vi "Init Device List.vi"(8 "error in (no error)":errorcluster, 9 "Active Devices":refnum<vi>, 10 "Subpanels' ref":refnum<vi>[](array[refnum])) -> (0 "error out":errorcluster, 2 "find list":string[](array[string]), 3 "Device List State out":T1)   [LabVIEW 2015]
uses:
  Device List State.ctl
  Device/Device.lvclass
  <vilib>/Instr/_visa.llb/VISA Find Search Mode.ctl
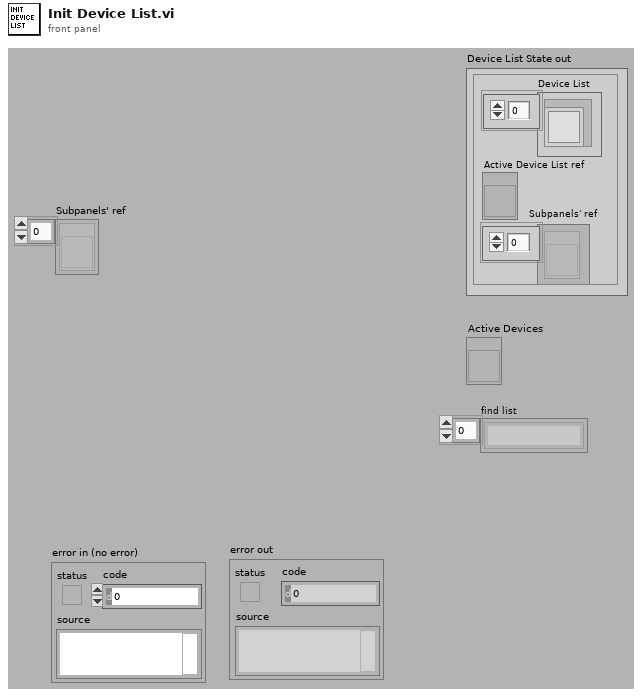
[diagram p1: front panel]
types:
  T1 = typedef "Device List State.ctl" = cluster{"Device List":refnum<class "Device.lvclass">[], "Active Device List ref":refnum<vi>, "Subpanels' ref":refnum<vi>[]}
  T2 = typedef "VISA Find Search Mode.ctl" = u32
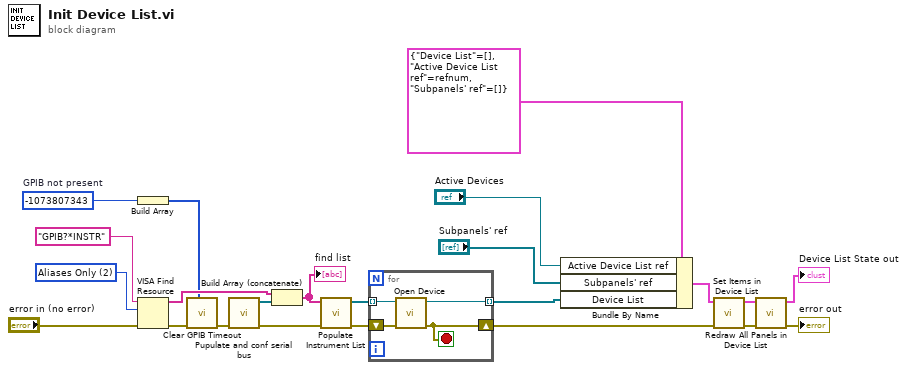
[diagram p0: block diagram]
diagram:
  w5 = -1073807343  # GPIB not present
  w22 = T2 2 items=["Canonical Names Only"=0, "Aliases Only"=2, "Include Matching Aliases"=3, "Include All Aliases"=4] ("Search Mode")
  n1 = Build Array(w5) -> (w4:i32[])
  n2 = VISA Find Resource(8:"error in (no error)", 10:w22, 11:"GPIB?*INSTR" ("expression (\"?*\")")) -> (0:w3:errorcluster, 3:w7:string[])  [unwired: 1 out]
  n3 = call "Clear GPIB Timeout.vi"("Errors to skip"=w4, "error in (no error)"=w3) -> ("error out"=w2:errorcluster)  [unwired: 9 out]
  n4 = call "Pupulate and conf serial bus.vi"("Error In"=w2) -> ("Error Out"=w1:errorcluster, "Devices"=w8:refnum<visa-resource-name>[])  [unwired: 9 in]
  n5 = Build Array (concatenate)(w7, w8) -> (w6:string[])
  "find list" <- w6
  n6 = call "Populate Instrument List.vi"("error in (no error)"=w1, "VISA Resourse Names"=w6) -> ("error out"=w20:errorcluster, "Instrument List"=w19:refnum<class "Instrument.lvclass">[])  [unwired: 2 in, 6 out]
  n7 = for {
    tunnel: w19 -> [w27] mode=indexing
    shift-right: [w24] -> w18
    shift-left: w20 -> [w25]
    tunnel: [w26] -> w11 mode=indexing
    stop <- w24 stop-if-true
    n8 = call "Open Device.vi"("error in (no error)"=w25, "Device"=w27) -> ("error out"=w24:errorcluster, "Device out"=w26:refnum<class "Instrument.lvclass">)  [unwired: 8 in]
  }
  n9 = Bundle By Name(cluster=T1 {"Device List"=[], "Active Device List ref"=refnum, "Subpanels' ref"=[]} ("Device List State out"), "Active Device List ref"="Active Devices", "Subpanels' ref"="Subpanels' ref", "Device List"=w11) -> (w14:T1)
  n10 = call "Set Items in Device List.vi"("Error In"=w18, "Device List State"=w14) -> ("Error Out"=w9:errorcluster, "Device List State out"=w13:T1)  [unwired: 8 in]
  n11 = call "Redraw All Panels in Device List.vi"("error in (no error)"=w9, "Device List State"=w13) -> ("error out"=→"error out":errorcluster, "Device List State out"=→"Device List State out":T1)  [unwired: 8 in]
